vi "launch_cRIO_VI.vi"() -> ()   [LabVIEW 2020]
panel:
  in  "stop":bool
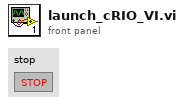
[diagram p1: front panel]
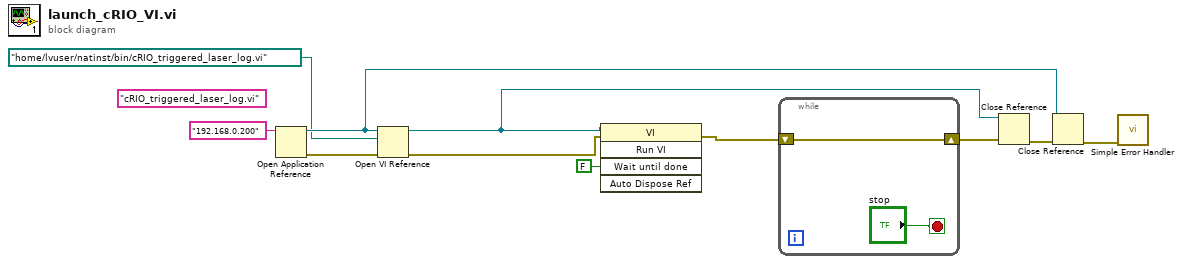
[diagram p0: block diagram]
diagram:
  (unwired) "cRIO_triggered_laser_log.vi" ("machine name (\"\":  open local reference)")
  n1 = Open Application Reference(11:"192.168.0.200" ("machine name (\"\":  open local reference)")) -> (0:w10:errorcluster, 3:w7:refnum<vi>)  [unwired: 3 in]
  n2 = Open VI Reference(application reference (local)=w7, vi path=path "/home/lvuser/natinst/bin/cRIO_triggered_laser_log.vi", error in (no error)=w10) -> (vi reference=w4:refnum<vi>, error out=w5:errorcluster)  [unwired: 3 in]
  n3 = invoke class="VI" method="Run VI"(reference=w4, error in=w5, "Wait until done"=FALSE ("Wait Until Done")) -> (error out=w2:errorcluster)  [unwired: 2 in, 4 out]
  n4 = while {
    shift-right: [w12] -> w9
    shift-left: w2 -> [w12]
    stop <- "stop" stop-if-true
  }
  n5 = Close Reference(reference=w4, error in (no error)=w9) -> (error out=w8:errorcluster)
  n6 = Close Reference(reference=w7, error in (no error)=w8) -> (error out=w6:errorcluster)
  n7 = call <vilib>:"Simple Error Handler.vi"("error in (no error)"=w6) -> ()  [unwired: 4 in, 5 out]
